vi "sender.vi"() -> ()   [LabVIEW 2019]
uses:
  <vilib>/httpClient/LabVIEWHTTPClient.lvlib
  <vilib>/smtpClient/LabVIEWSMTPClient.lvlib
panel:
  in  "?":bool
  in  "url":string
  in  "Push":bool
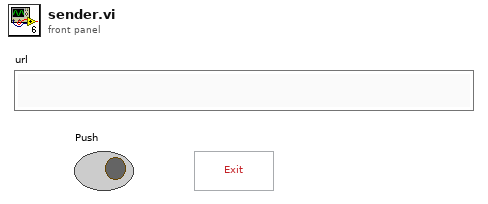
[diagram p1: front panel]
types:
  T1 = typedef "LabVIEWHTTPClient.lvlib/ClientHandle.ctl" = refnum<k1>
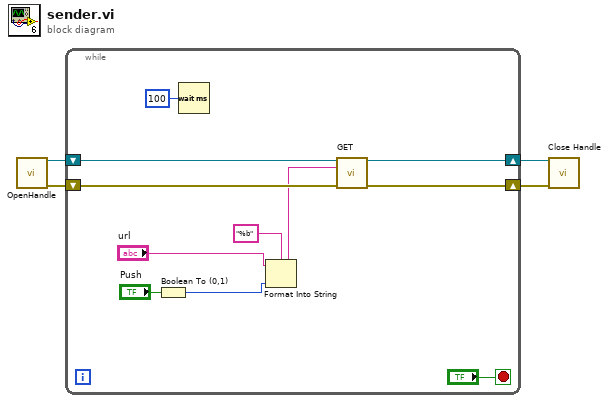
[diagram p0: block diagram]
diagram:
  n1 = call <vilib>:"OpenHandle.vi"() -> ("client handle out"=w4:T1, "error out"=w2:errorcluster)  [unwired: 14 in]
  n2 = while {
    shift-right: [w14] -> w3
    shift-left: w4 -> [w15]
    shift-right: [w12] -> w1
    shift-left: w2 -> [w13]
    stop <- "?" stop-if-true
    n3 = Boolean To (0,1)(Boolean="Push") -> (0, 1=w9:i16)
    n4 = Wait (ms)(milliseconds to wait=u32 100) -> ()  [unwired: 1 out]
    n5 = Format Into String(format string="%b", initial string="url", w9) -> (resulting string=w7:string)  [unwired: 1 in, 1 out]
    n6 = call <vilib>:"GET.vi"("client handle"=w15, "url"=w7, "error in (no error)"=w13) -> ("client handle out"=w14:T1, "error out"=w12:errorcluster)  [unwired: 9 in, 2 out]
  }
  n7 = call <vilib>:"Close Handle.vi"("handle in"=w3, "error in (no error)"=w1) -> ()  [unwired: 12 in, 2 out]
